vi "Sort RD Data.vi"(2 "rawRD":i16[][][](array[numeric]), 3 "rd_fit":bool, 4 "rd_sel":bool[](array[boolean]), 5 "rd_data":bool) -> (0 "Res":sgl[][](array[numeric]), 1 "rd&RdFit":sgl[][](array[numeric]))   [LabVIEW 2012]
doc: "Sort the ringdown data so that the ringdowns, fits and residuals are plotted properly."
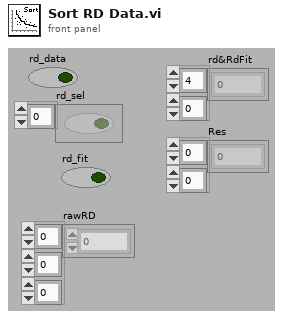
[diagram p1: front panel]
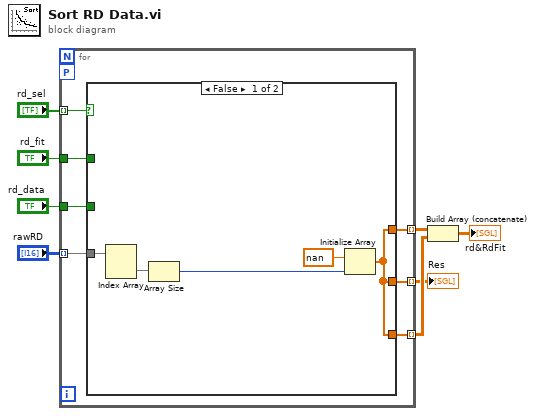
[diagram p0: block diagram]
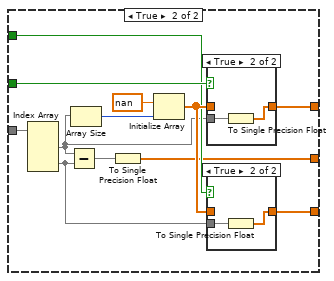
[diagram p2: hidden frame]
diagram:
  n1 = for {
    tunnel: "rd_sel" -> [w15] mode=indexing
    tunnel: [w14] -> w5 mode=indexing
    tunnel: [w13] -> w4 mode=indexing
    tunnel: [w12] -> w3 mode=indexing
    workers-P: _ -> [_]
    tunnel: "rd_data" -> [w11]
    tunnel: "rd_fit" -> [w10]
    tunnel: "rawRD" -> [w9] mode=indexing
    n2 = case shown="False" w15 {
      tunnel: [w18 w30] -> w14
      tunnel: [w18 w29] -> w13
      tunnel: [w18 w21] -> w12
      tunnel: w11 -> [_ w27]
      tunnel: w10 -> [_ w26]
      tunnel: w9 -> [w17 w25]
      frame False {
        n3 = Index Array(array=w17) -> (element=w16:i16[])  [unwired: 2 in]
        n4 = Array Size(array=w16) -> (size(s)=w20:i32)
        n5 = Initialize Array(sgl nan ("element"), w20) -> (w18:sgl[])
      }
      frame True {
        n6 = Index Array(array=w25) -> (element #1=w24:i16[], element #2=w23:i16[])  [unwired: 4 in]
        n7 = Subtract(x=w24, y=w23) -> (x-y=w22:i16[])
        n8 = Array Size(array=w24) -> (size(s)=w31:i32)
        n9 = To Single Precision Float(number=w22) -> (single precision float=w21:sgl[])
        n10 = Initialize Array(sgl nan ("element"), w31) -> (w28:sgl[])
        n11 = case shown="True" w27 {
          tunnel: w28 -> [w36 _]
          tunnel: [w36 w37] -> w30
          tunnel: w24 -> [_ w38]
          frame False {
          }
          frame True {
            n12 = To Single Precision Float(number=w38) -> (single precision float=w37:sgl[])
          }
        }
        n13 = case shown="True" w26 {
          tunnel: [w33 w34] -> w29
          tunnel: w23 -> [_ w35]
          tunnel: w28 -> [w33 _]
          frame False {
          }
          frame True {
            n14 = To Single Precision Float(number=w35) -> (single precision float=w34:sgl[])
          }
        }
      }
    }
  }
  "Res" <- w3
  n15 = Build Array (concatenate)(w5, w4) -> (→"rd&RdFit":sgl[][])
